vi "Init.vi"(8 "error in (no error)":errorcluster, 11 "reference in":refnum<class "Flux_Capacitor.lvclass">) -> (0 "error out":errorcluster, 3 "reference out":refnum<class "Flux_Capacitor.lvclass">)   [LabVIEW 2022 SP3, in "Flux_Capacitor.lvlib" / "Flux_Capacitor.lvclass"]
uses:
  Flux_Capacitor.lvclass
  TempSensor.ctl
  <vilib>/numeric/Random Number (Range) U64.vi
  <vilib>/numeric/sub_Random U32.vi
  Components/ViPER.lvlibp/ViPER.lvclass
  C:/Projects/Medulla/ViPER/Examples/Flux_Capacitor_Tester/Components/ViPER.lvlibp/ViPER.lvclass
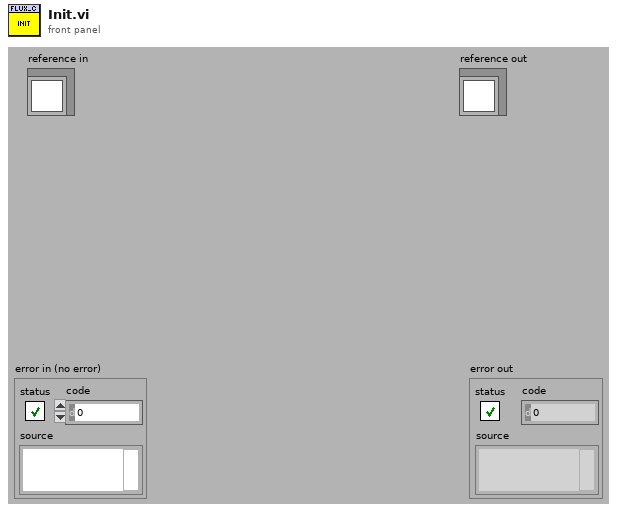
[diagram p1: front panel]
types:
  T1 = typedef "Flux_Capacitor.lvlib/Flux_Capacitor.lvclass/TempSensor.ctl" = enum16{"1", "2", "3"}
  T2 = typedef "Flux_Capacitor.lvlib/Flux_Capacitor.lvclass/ObjectAttributes.ctl" = cluster{"Config":T3, "T Sensors":T1[], "Temp_DegC":dbl[], "Temp_Raw":u64[], "RTC":timestamp, "Flux":bool, "Time":timestamp, "RTC_Live":timestamp}
  T3 = typedef "Flux_Capacitor.lvlib/Flux_Capacitor.lvclass/Config.ctl" = cluster{"default":string}
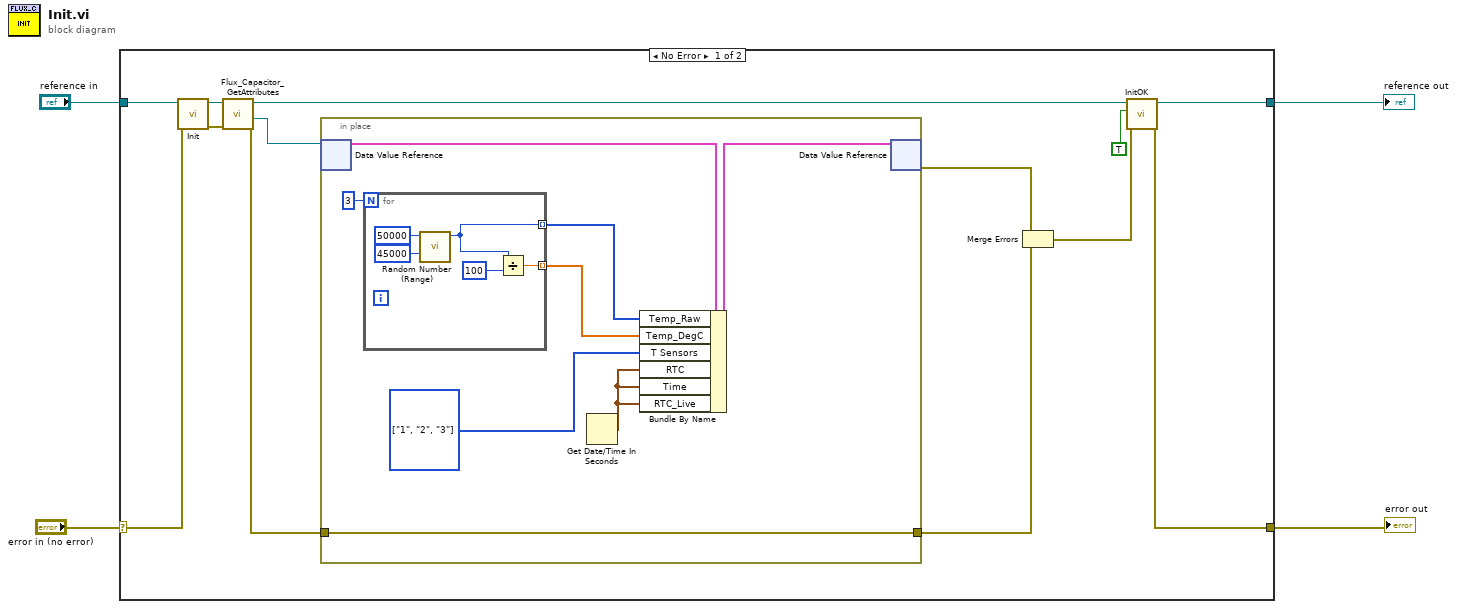
[diagram p0: block diagram]
diagram:
  n1 = case shown="No Error" "error in (no error)" {
    selector: "error in (no error)" -> [w16 w32]
    tunnel: [w9 w32] -> w3
    tunnel: [w10 w31] -> w1
    tunnel: "reference in" -> [w17 w31]
    frame No Error {
      n2 = call-parent "Init.vi"("error in (no error)"=w16, "reference in"=w17) -> ("error out"=w14:errorcluster, "reference out"=w15:refnum<class "Flux_Capacitor.lvclass">)  [unwired: 8 in]
      n3 = call "Flux_Capacitor_GetAttributes.vi"("error in (no error)"=w14, "reference in"=w15) -> ("error out"=w12:errorcluster, "DataRef"=w13:refnum<data-value>, "reference out"=w5:refnum<class "Flux_Capacitor.lvclass">)  [unwired: 6 in, 1 out]
      n4 = in-place {
        in-place-border: w12 -> [w23]
        in-place-border: [w23] -> w8
        w22 = T1[] [enum."1", enum."2", enum."3"] items=["1", "2", "3"] ("T Sensors")
        n5 = in-place-dvr #1(w13) -> (w25:T2)  [unwired: 1 out]
        n6 = for {
          N: 3 -> [_]
          tunnel: [w26] -> w20 mode=indexing
          tunnel: [w28] -> w19 mode=indexing
          n7 = call-poly <vilib>:"Random Number (Range).vi"("lower bound (0)"=u64 45000, "upper bound (100)"=u64 50000) -> ("number"=w28:u64)  [unwired: 9 in]
          n8 = Divide(x=w28, y=u64 100) -> (x/y=w26:dbl)
        }
        n9 = Get Date/Time In Seconds() -> (seconds since 1Jan1904=w18:timestamp)
        n10 = Bundle By Name(cluster=w25, "Temp_Raw"=w19, "Temp_DegC"=w20, "T Sensors"=w22, "RTC"=w18, "Time"=w18, "RTC_Live"=w18) -> (w24:T2)
        n11 = in-place-dvr #1(w24) -> (w6:errorcluster)  [unwired: 1 out]
      }
      n12 = Merge Errors(w6, w8) -> (w7:errorcluster)
      n13 = call "InitOK.vi"("error in (no error)"=w7, "Init OK?"=TRUE, "reference in"=w5) -> ("error out"=w9:errorcluster, "reference out"=w10:refnum<class "Flux_Capacitor.lvclass">)  [unwired: 7 in]
    }
    frame Error {
    }
  }
  "error out" <- w3
  "reference out" <- w1
